vi "configUI.vi"() -> ()   [LabVIEW 2017, in "ActiveFrontEndModule editor node.lvclass"]
doc: "All child modules share this same UI. The UI allows for the configuration of Channels, Parameters, and Error Handling."
uses:
  ActiveFrontEndModule editor node.lvclass
  <vilib>/NI/Configuration Framework/Node/NodeRef.ctl
  <vilib>/NI/Configuration Framework/Node/NISE_CEF_Node.lvclass
  <vilib>/NI/AMC/Message Queue.ctl
  <vilib>/NI/AMC/Message.ctl
  <vilib>/NI/Tools/Keyed Array/KeyedArray.ctl
  <vilib>/NI/Configuration Framework/Node/UserEventRef.ctl
  <vilib>/NI/Configuration Framework/Controls/EventCluster.ctl
  <vilib>/NI/DCAF/Tag Editor Core/control module/configuration/error classification setting.ctl
  <vilib>/NI/Tag Bus Module Framework/runtime/error classification.ctl
  <vilib>/NI/Configuration Framework/Node/RefreshUIEvent.ctl
  <vilib>/NI/Configuration Framework/Node/CacheState.ctl
  <vilib>/NI/Configuration Framework/Node/StopEvent.ctl
  <vilib>/NI/Configuration Framework/Node/NodeChangeEvent.ctl
  <vilib>/NI/DCAF/Tag Editor Core/Table API/Available Tag Menu/channel action event.ctl
  <vilib>/NI/DCAF/Tag Editor Core/Table API/Available Tag Menu/dialog output action.ctl
  <vilib>/NI/Tag Bus Module Framework/channel/TBM channel.lvclass
  <vilib>/NI/Tag Bus/tag/tag descriptor.lvclass
  <vilib>/NI/DCAF/Tag Editor Core/Table API/Table Manager/Call Back Ref Type Def.ctl
  <vilib>/NI/DCAF/Tag Editor Core/Configuration Editor/Classes/Engine Parent/Engine Parent Editor Node.lvclass
  <vilib>/NI/DCAF/Tag Editor Core/Configuration Editor/Classes/Module editor node/module editor node.lvclass
  C:/Program Files (x86)/National Instruments/LabVIEW 2017/vi.lib/NI/Configuration Framework/serializable node/NISE_CEF_serializable node.lvclass
  <vilib>/NI/PowerElectronicsControl/ActiveFrontEnd/AFE/PI_Settings.ctl
  <vilib>/rvi/Analysis/control/PID/Typedef/niFpgaPID_PIGains.ctl
  <vilib>/rvi/Analysis/control/PID/Typedef/niFpgaPID_OutputRange.ctl
  <vilib>/NI/PowerElectronicsControl/ActiveFrontEnd/AFE/Parameters.ctl
  <vilib>/NI/PowerElectronicsControl/ActiveFrontEnd/AFE/Mode.ctl
  <vilib>/NI/DCAF/Tag Editor Core/Table API/Table Manager/references.ctl
  <vilib>/NI/DCAF/Tag Editor Core/Table API/Table Manager/Menu Definition.ctl
  <vilib>/NI/DCAF/Tag Editor Core/Table API/Table Manager/Menu Options.ctl
  <vilib>/NI/DCAF/Tag Editor Core/control module/configuration/control module configuration.lvclass
  C:/Program Files (x86)/National Instruments/LabVIEW 2017/vi.lib/NI/Configuration Framework/serializable configuration/NISE_CEF_serializable configuration.lvclass
  <vilib>/NI/DCAF/Tag Editor Core/control module/editor node/control module editor.lvclass
  C:/Program Files (x86)/National Instruments/LabVIEW 2017/vi.lib/NI/DCAF/Tag Editor Core/Configuration Editor/Classes/Module editor node/module editor node.lvclass
  module/configuration/ActiveFrontEndModule configuration.lvclass
  C:/Program Files (x86)/National Instruments/LabVIEW 2017/vi.lib/NI/DCAF/Tag Editor Core/control module/configuration/control module configuration.lvclass
  C:/Program Files (x86)/National Instruments/LabVIEW 2017/vi.lib/NI/Tag Bus Module Framework/module configuration/TBM module configuration.lvclass
  module/configuration/ActiveFrontEndModule configuration.lvclass/ActiveFrontEndModule configuration.ctl
  <vilib>/NI/DCAF/Tag Editor Core/control module/configuration/control module configuration.lvclass/control module configuration.ctl
  <vilib>/NI/Configuration Framework/serializable configuration/NISE_CEF_serializable configuration.lvclass/NISE_CEF_serializable configuration.ctl
  <vilib>/NI/Tag Bus Module Framework/channel/channel classification.ctl
  module/configuration/Read ID_to_VD.vi
  module/configuration/Read IQ_to_VQ.vi
  module/configuration/Read VDCLinkToPower.vi
  module/configuration/Read Parameters.vi
  module/configuration/Write VDCLinkToPower.vi
  module/configuration/Write ID_to_VD.vi
  module/configuration/Write IQ_to_VQ.vi
  module/configuration/Write Parameters.vi
  <vilib>/NI/DCAF/Tag Editor Core/control module/configuration/Write error classifications.vi
  <vilib>/NI/Tag Bus Module Framework/module configuration/TBM module configuration.lvclass
  <vilib>/NI/DCAF/Tag Editor Core/Configuration Editor/Classes/Module editor node/Read Module Configuration.vi
  <vilib>/NI/DCAF/Tag Editor Core/control module/editor node/read fixed channel configuration.vi
  <vilib>/NI/DCAF/Tag Editor Core/Configuration Editor/Classes/Module editor node/Write Module Configuration.vi
  <vilib>/Utility/LVClass/Get LV Class Name.vi
  <vilib>/NI/Configuration Framework/error generator/NISE_error generator.vi
  <vilib>/NI/Configuration Framework/serializable configuration/NISE_CEF_serializable configuration.lvclass
  <vilib>/NI/DCAF/Tag Editor Core/Table API/Listbox/Multi Column Listbox.lvclass
  <vilib>/NI/Configuration Framework/NISE_CEF_TreeControl.lvlib
  <vilib>/NI/DCAF/Tag Editor Core/Table API/Table Manager.lvlib
  <vilib>/NI/DCAF UI Toolkit/Controls/DCAF UI Elements.lvlib
  <vilib>/NI/Tools/Keyed Array/Tools_KeyedArray.lvlib
  <vilib>/NI/AMC/AMC.lvlib
  <vilib>/NI/DCAF/Tag Editor Core/Table API/Table Manager/Table Manager.lvclass
  <vilib>/NI/Tag Bus Module Framework/runtime/TBM module execution interface.lvclass
  <vilib>/NI/PowerElectronicsControl/ActiveFrontEnd/AFE/ActiveFrontEnd.lvlib
panel:
  in  "Enum":i32
  in  "user event out":refnum<user-event>
  in  "Top Level Tab Control":T1(tab)
  in  "ID_to_VD":T2={"gains"={"proportional gain"=0.0, "integral gain"=0.0}, "output range"={"output high (Inf)"=inf, "output low (-Inf)"=-inf}, "PI_state"=enum."idle", "reset"=FALSE, "manual"=0.0} {"gains"."proportional gain" step=0.125}
  in  "IQ_to_VQ":T2={"gains"={"proportional gain"=0.0, "integral gain"=0.0}, "output range"={"output high (Inf)"=inf, "output low (-Inf)"=-inf}, "PI_state"=enum."idle", "reset"=FALSE, "manual"=0.0} {"gains"."proportional gain" step=0.125}
  in  "VDCLinkToPower":T2={"gains"={"proportional gain"=0.0, "integral gain"=0.0}, "output range"={"output high (Inf)"=inf, "output low (-Inf)"=-inf}, "PI_state"=enum."idle", "reset"=FALSE, "manual"=0.0} {"gains"."proportional gain" step=0.125}
  in  "Initial Parameters":T5
  in  "Channels Listbox":i32(listbox)
  in  "mapall":bool
  in  "mapwriters":bool
  in  "Parameters Listbox":i32(listbox)
  in  "error classifications":T7[](array[typedef])
  in  "node change":T9
  in  "stop event":T10
  in  "cache state":T11
  in  "refresh UI":T12
  in  "user event":T13
  in  "main queue":T14
  in  "node ref":T15
  # "(Single-Click to Edit)"
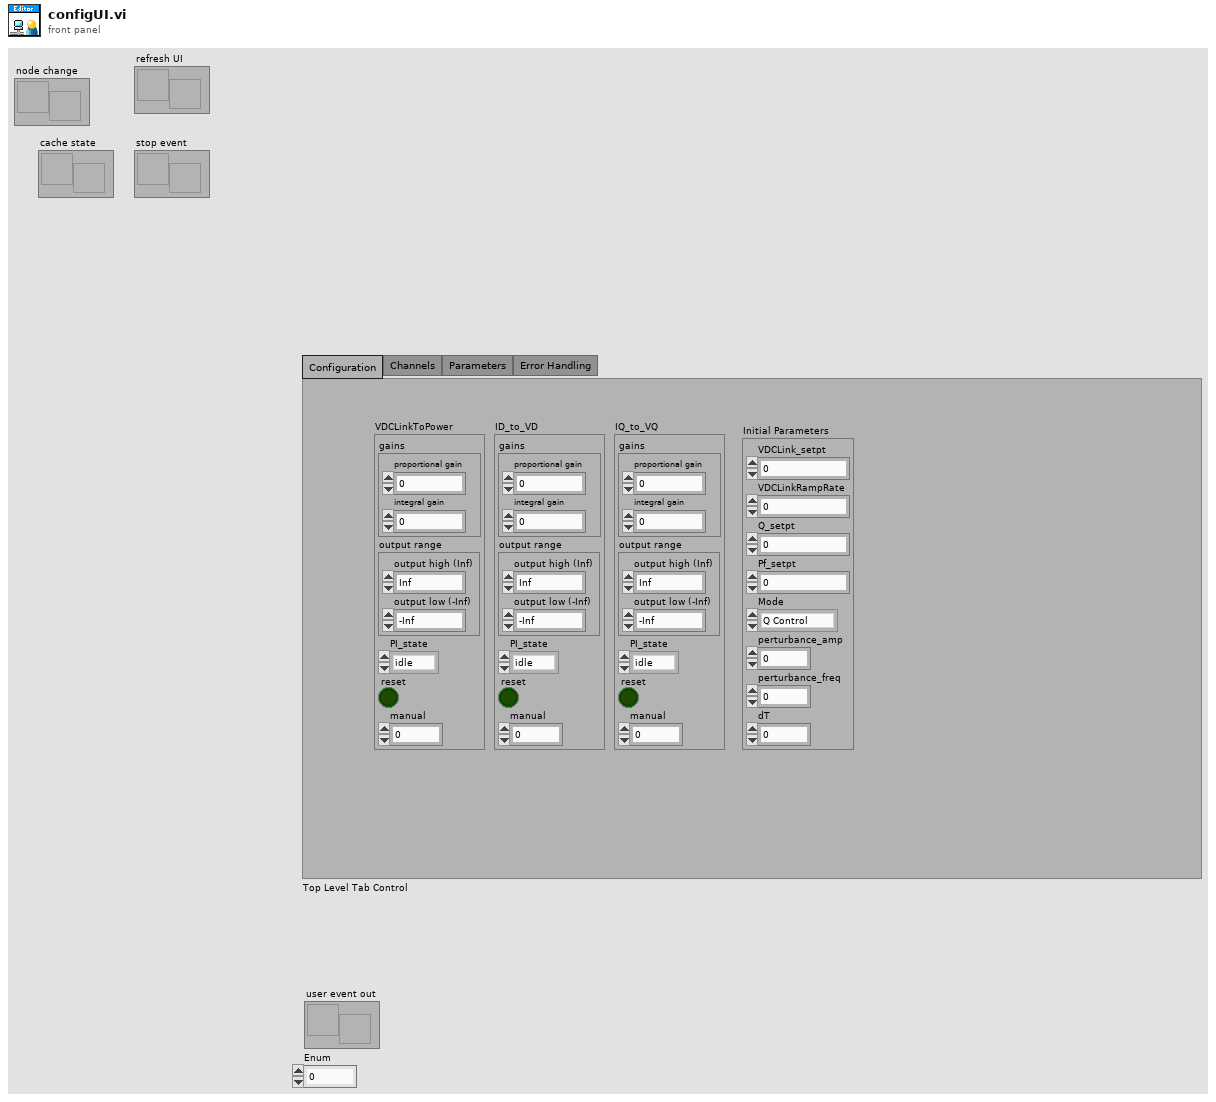
[diagram p1: front panel]
types:
  T1 = enum32{"Configuration", "Channels", "Parameters", "Error Handling"}
  T2 = typedef "ActiveFrontEnd.lvlib/PI_Settings.ctl" = cluster{"gains":T3, "output range":T4, "PI_state":enum8{"idle", "normal", "manual", "perturbance"}, "reset":bool, "manual":sgl}
  T3 = typedef "niFpgaPID_PIGains.ctl" = cluster{"proportional gain":sgl, "integral gain":sgl}
  T4 = typedef "niFpgaPID_OutputRange.ctl" = cluster{"output high (Inf)":sgl, "output low (-Inf)":sgl}
  T5 = typedef "ActiveFrontEnd.lvlib/Parameters.ctl" = cluster{"VDCLink_setpt":sgl, "VDCLinkRampRate":sgl, "Q_setpt":sgl, "Pf_setpt":sgl, "Mode":T6, "perturbance_amp":sgl, "perturbance_freq":sgl, "dT":sgl}
  T6 = typedef "ActiveFrontEnd.lvlib/Mode.ctl" = enum16{"Q Control", "Pf Control"}
  T7 = typedef "control module configuration.lvclass/error classification setting.ctl" = cluster{"code":i32, "error classification":T8}
  T8 = typedef "TBM module execution interface.lvclass/error classification.ctl" = enum16{"unknown", "none", "trivial", "recoverable", "critical"}
  T9 = typedef "NISE_CEF_Node.lvclass/NodeChangeEvent.ctl" = refnum<user-event>
  T10 = typedef "NISE_CEF_Node.lvclass/StopEvent.ctl" = refnum<user-event>
  T11 = typedef "NISE_CEF_Node.lvclass/CacheState.ctl" = refnum<user-event>
  T12 = typedef "NISE_CEF_Node.lvclass/RefreshUIEvent.ctl" = refnum<user-event>
  T13 = typedef "NISE_CEF_Node.lvclass/UserEventRef.ctl" = refnum<user-event>
  T14 = typedef "AMC.lvlib/Message Queue.ctl" = refnum<queue>
  T15 = typedef "NISE_CEF_Node.lvclass/NodeRef.ctl" = refnum<data-value>
  T16 = typedef "Table Manager.lvlib/Table Manager.lvclass/Menu Definition.ctl" = cluster{"Menu Name":string, "Menu Options":T17}
  T17 = typedef "Table Manager.lvlib/Table Manager.lvclass/Menu Options.ctl" = enum16{"Always Show", "Show When Used", "Show When Empty"}
  T18 = typedef "Table Manager.lvlib/Table Manager.lvclass/references.ctl" = cluster{"stop event":T10, "refresh UI":T12, "cache state":T11, "node change":T9, "user event out":refnum<user-event>, "main queue":T14, "user event":T13}
  T19 = typedef "Table Manager.lvlib/Column.lvclass/Column Descriptor.ctl" = cluster{"name":string, "caption":string, "Column Type":T20, "Params":string, "AutoSizeMode":i32, "FillWeight":sgl, "MinWidth":u32, "tooltip":string, "Enum Reference":refnum<vi>, "Channel suffix":string, "Read Only":bool, "Call Back VI":T21, "DT Dependency":i32, "name dependency":i32, "data type":T22, "Custom Column":refnum<class "Column.lvclass">}
  T20 = typedef "Table Manager.lvlib/Column.lvclass/Column Type.ctl" = enum16{"String", "Mapping", "Enum", "Custom"}
  T21 = typedef "Table Manager.lvlib/Table Manager.lvclass/Call Back Ref Type Def.ctl" = refnum<vi>
  T22 = typedef "tag bus.lvlib/tag descriptor.lvclass/Data Type.ctl" = enum16{"Double", "Single", "I64", "I32", "I16", "I8", "U64", "U32", "U16", "U8", "Boolean", "String", "Array of Double", "Array of Single", "Array of I64", "Array of I32", "Array of I16", "Array of I8", "Array of U64", "Array of U32", "Array of U16", "Array of U8", "Array of Boolean", "Array of String"}
  T23 = typedef "Table Manager.lvlib/Table Manager.lvclass/object ref.ctl" = cluster{"engine":refnum<data-value>, "Node Ref":refnum<data-value>}
  T24 = typedef "Table Manager.lvlib/Table Manager.lvclass/Table Events.ctl" = cluster{"Menu Selection":refnum<user-event>}
  T25 = typedef "NISE_CEF_TreeControl.lvlib/EventCluster.ctl" = cluster{"command":string, "data":string}
  T26 = typedef "TBM channel.lvclass/channel classification.ctl" = enum16{"input data", "output data", "processing parameter", "processing result"}
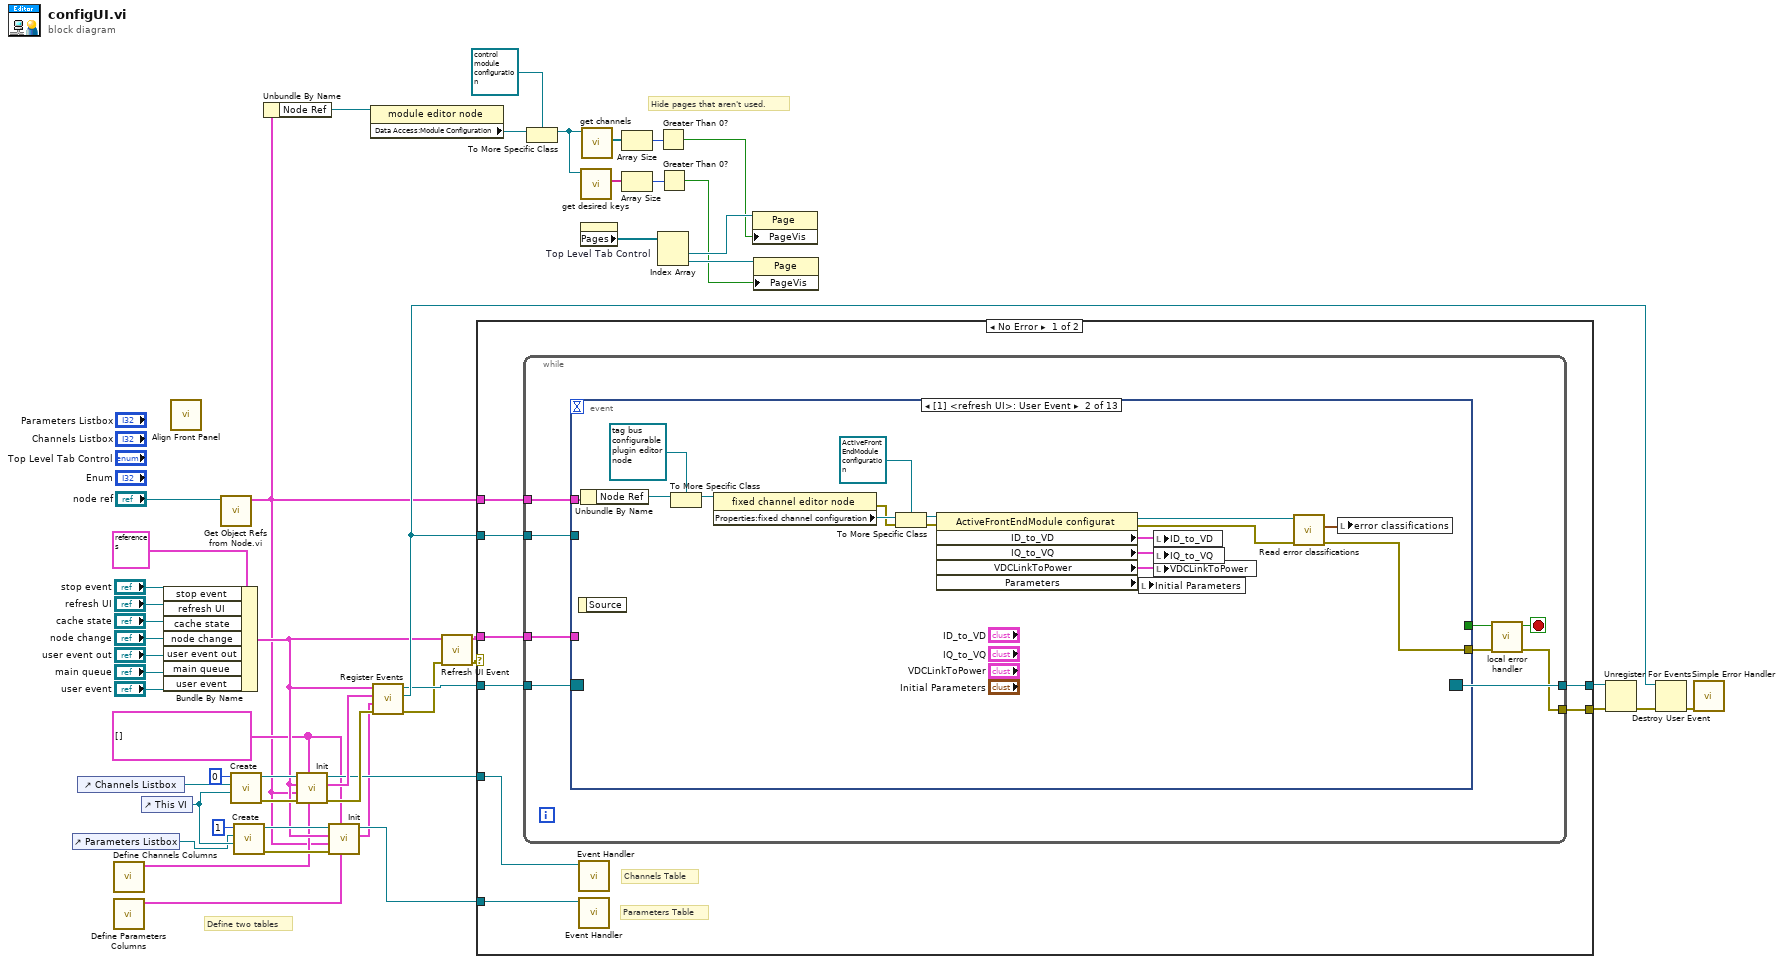
[diagram p0: block diagram]
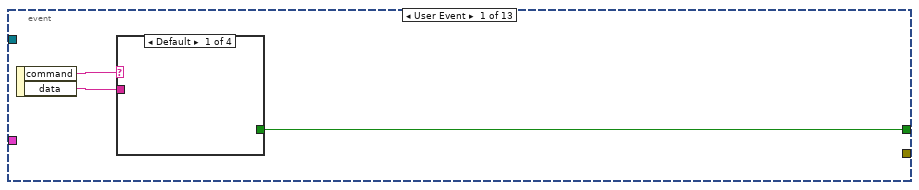
[diagram p2: hidden frame]
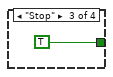
[diagram p4: hidden frame]
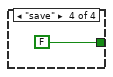
[diagram p5: hidden frame]
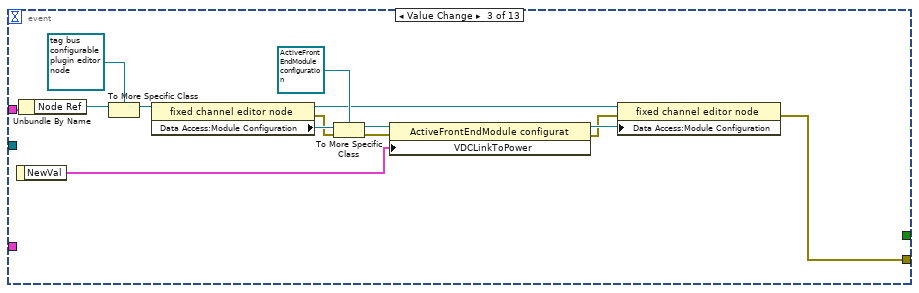
[diagram p6: hidden frame]
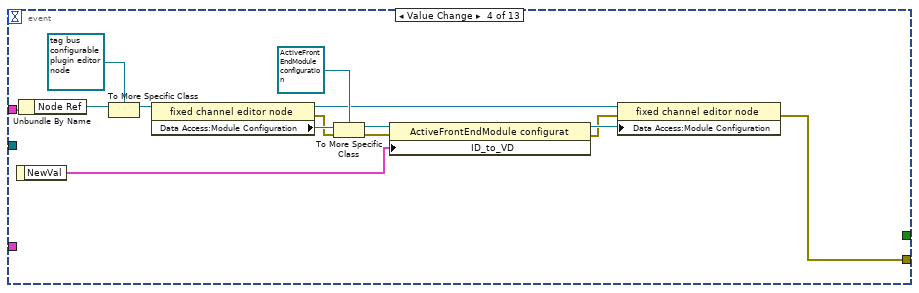
[diagram p7: hidden frame]
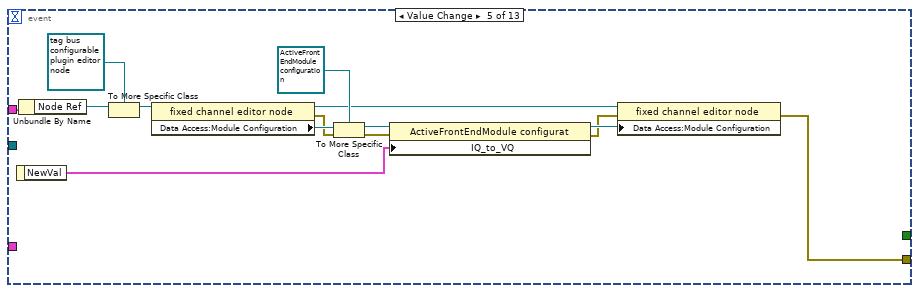
[diagram p8: hidden frame]
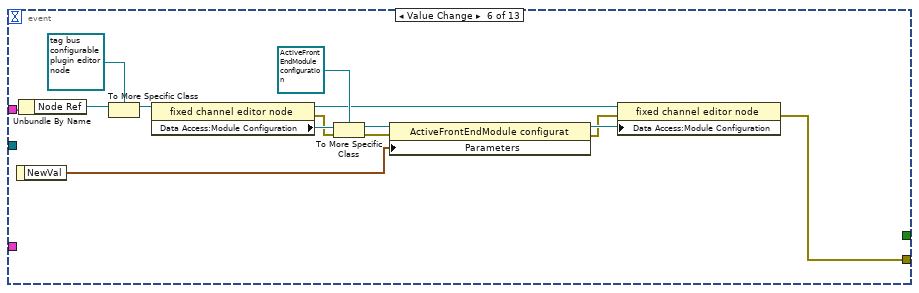
[diagram p9: hidden frame]
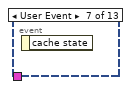
[diagram p10: hidden frame]
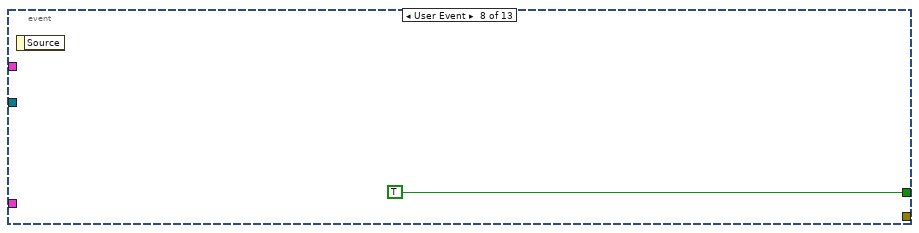
[diagram p11: hidden frame]
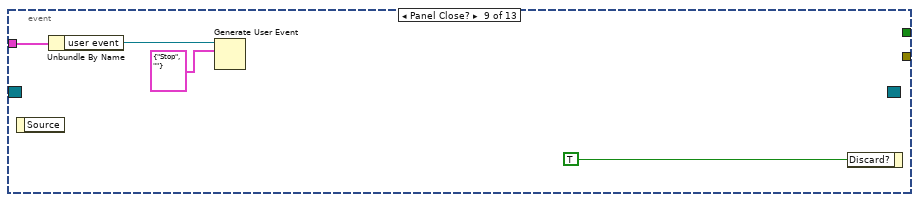
[diagram p12: hidden frame]
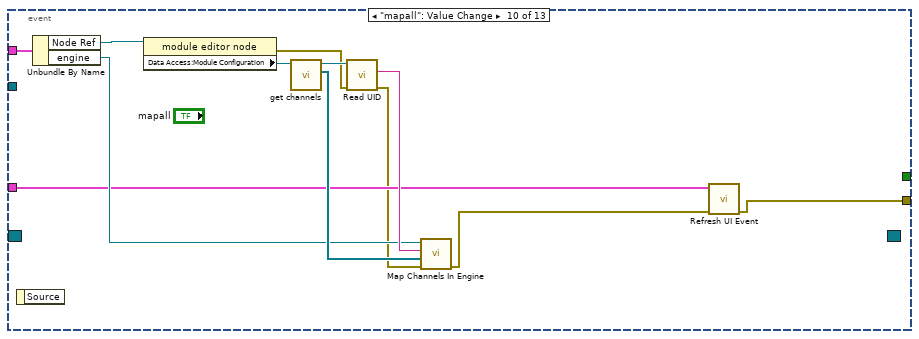
[diagram p13: hidden frame]
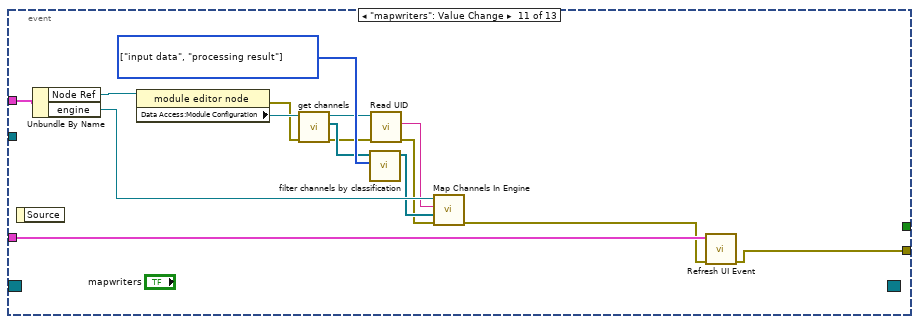
[diagram p14: hidden frame]
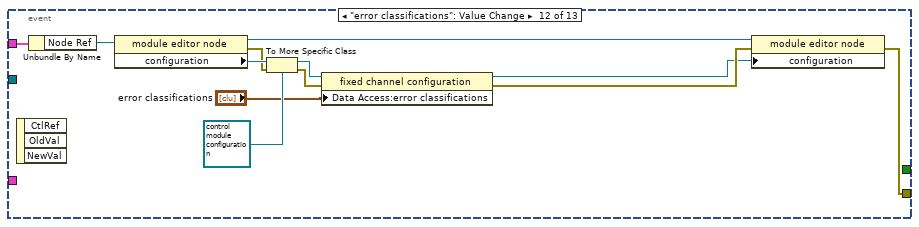
[diagram p15: hidden frame]
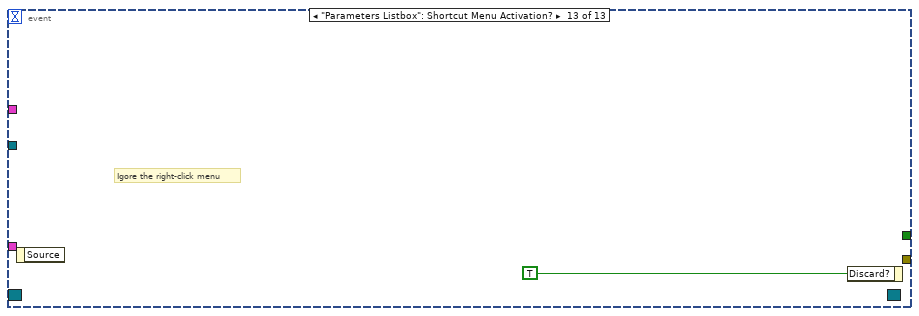
[diagram p16: hidden frame]
diagram:
  w15 = T16[] [] ("Right-Click Menu")
  # "Define two tables"
  # "Hide pages that aren't used."
  n1 = control-ref of="Parameters Listbox"() -> (w18:refnum<vi>)
  n2 = control-ref of="Channels Listbox"() -> (w26:refnum<vi>)
  n3 = call <vilib>:"Define Channels Columns.vi"() -> ("Column Descriptors"=w17:T19[])  [unwired: 11 in]
  n4 = call <vilib>:"Define Parameters Columns.vi"() -> ("Column Descriptors"=w16:T19[])  [unwired: 11 in]
  n5 = control-ref of="This VI"() -> (w22:refnum<vi>)
  n6 = Bundle By Name(cluster=T18 {"stop event"=refnum, "refresh UI"=refnum, "cache state"=refnum, "node change"=refnum, "user event out"=refnum, "main queue"=refnum, "user event"=refnum} ("Event References"), "stop event"="stop event", "refresh UI"="refresh UI", "cache state"="cache state", "node change"="node change", "user event out"="user event out", "main queue"="main queue", "user event"="user event") -> (w19:T18)
  n7 = call <vilib>:"Align Front Panel.vi"() -> ()  [unwired: 10 in, 2 out]
  n8 = call <vilib>:"Get Object Refs from Node.vi.vi"("node ref"="node ref") -> ("Node object refs"=w7:T23)  [unwired: 9 in, 1 out]
  n9 = call <vilib>:"Create.vi"("Top VI"=w22, "Listbox"=w26, "Index"=0) -> ("error out"=w29:errorcluster, "reference out"=w30:refnum<class "Multi Column Listbox.lvclass">)  [unwired: 7 in]
  n10 = call <vilib>:"Create.vi"("Top VI"=w22, "Listbox"=w18, "Index"=1) -> ("error out"=w25:errorcluster, "reference out"=w24:refnum<class "Multi Column Listbox.lvclass">)  [unwired: 7 in]
  n11 = Unbundle By Name(w7) -> ("Node Ref"=w5:refnum<data-value>)
  n12 = call-dynamic "Init.vi"("Column Descriptors"=w17, "Right-Click Menu"=w15, "error in (no error)"=w29, "Node object refs"=w7, "Event References"=w19, "Multi Column Listbox in"=w30) -> ("error out"=w28:errorcluster, "Table Events"=w40:T24, "Multi Column Listbox out"=w27:refnum<class "Multi Column Listbox.lvclass">)  [unwired: 3 in]
  n13 = call-dynamic "Init.vi"("Column Descriptors"=w16, "Right-Click Menu"=w15, "error in (no error)"=w25, "Node object refs"=w7, "Event References"=w19, "Multi Column Listbox in"=w24) -> ("Table Events"=w20:T24, "Multi Column Listbox out"=w21:refnum<class "Multi Column Listbox.lvclass">)  [unwired: 3 in, 1 out]
  n14 = property class="module editor node"(reference=w5) -> ("Data Access:Module Configuration"=w6:refnum<class "TBM module configuration.lvclass">)  [unwired: 1 in, 2 out]
  n15 = call <vilib>:"Register Events.vi"("error in (no error)"=w28, "Parameters Table Events"=w20, "Channels Table Events"=w40, "Event References"=w19) -> ("error out"=w33:errorcluster, "Channel Action"=w39:refnum<user-event>, "Event Registration Refnum"=w38:refnum<event-registration>)  [unwired: 5 in]
  n16 = call <vilib>:"Refresh UI Event.vi"("error in (no error)"=w33, "Event References"=w19) -> ("error out"=w34:errorcluster, "Event References out"=w32:T18)  [unwired: 8 in]
  n17 = case shown="No Error" w34 {
    selector: w34 -> [_ w191]
    tunnel: w38 -> [w58 w190]
    tunnel: [w57 w190] -> w50
    tunnel: [w55 w191] -> w49
    tunnel: w39 -> [w56 _]
    tunnel: w7 -> [w54 _]
    tunnel: w32 -> [w53 _]
    tunnel: w27 -> [w52 _]
    tunnel: w21 -> [w51 _]
    frame No Error {
      # "Parameters Table"
      # "Channels Table"
      n18 = while {
        tunnel: w58 -> [w67]
        tunnel: [w66] -> w57
        tunnel: w56 -> [w65]
        tunnel: [w61] -> w55
        tunnel: w54 -> [w60]
        tunnel: w53 -> [w59]
        stop <- w63 stop-if-true
        n19 = event shown="[1] <refresh UI>: User Event" {
          selector: w67 -> [_ _ _ _ _ _ _ _ _ _ _ _ _]
          dyn-events: [_ _ _ _ _ _ _ _ _ _ _ _ _] -> w66
          timeout: _ -> [_ _ _ _ _ _ _ _ _ _ _ _ _]
          tunnel: [w70 _ _ _ _ _ _ TRUE _ _ _ _ _] -> w64
          tunnel: [_ w86 w91 w105 w119 w133 _ _ _ w156 w172 w188 _] -> w62
          tunnel: w65 -> [_ _ _ _ _ _ _ _ _ _ _ _ _]
          tunnel: w60 -> [_ w89 w103 w117 w131 w145 _ _ _ w160 w173 w187 _]
          tunnel: w59 -> [_ _ _ _ _ _ _ _ w148 w155 w171 _ _]
          event User Event {
            n20 = event-data() -> ("command"=w69:string, "data"=w68:string)  [unwired: 1 in]
            n21 = case shown="Default" w69 {
              tunnel: [_ _ TRUE FALSE] -> w70
              tunnel: w68 -> [_ _ _ _]
              frame Default {
              }
              frame "Refresh" {
              }
              frame "Stop" {
              }
              frame "save" {
              }
            }
          }
          event User Event {
            n22 = event-data() -> ()  [unwired: 1 in, 1 out]
            n23 = Unbundle By Name(w89) -> ("Node Ref"=w87:refnum<data-value>)
            n24 = To More Specific Class(target class=refnum<data-value> refnum ("data value reference"), reference=w87) -> (specific class reference=w85:refnum<data-value>)  [unwired: 1 in, 1 out]
            n25 = property class="fixed channel editor node"(reference=w85) -> (error out=w82:errorcluster, "Properties:fixed channel configuration"=w83:refnum<class "control module configuration.lvclass">)  [unwired: 1 in, 1 out]
            n26 = To More Specific Class(target class=refnum<class "ActiveFrontEndModule configuration.lvclass"> refnum ("ActiveFrontEndModule configuration"), reference=w83, error in=w82) -> (specific class reference=w80:refnum<class "ActiveFrontEndModule configuration.lvclass">, error out=w78:errorcluster)
            n27 = property class="ActiveFrontEndModule configurat"(reference=w80, error in=w78) -> (reference out=w79:refnum<class "ActiveFrontEndModule configuration.lvclass">, error out=w77:errorcluster, "ID_to_VD"=w76:T2, "IQ_to_VQ"=w75:T2, "VDCLinkToPower"=w74:T2, "Parameters"=w73:T5)
            n28 = local write "Initial Parameters"(w73) -> ()
            n29 = local write "ID_to_VD"(w76) -> ()
            n30 = local write "IQ_to_VQ"(w75) -> ()
            n31 = local write "VDCLinkToPower"(w74) -> ()
            n32 = call <vilib>:"Read error classifications.vi"("error in"=w77, "control module configuration in"=w79) -> ("error out"=w86:errorcluster, "error classifications"=w84:T7[])  [unwired: 7 in, 1 out]
            n33 = local write "error classifications"(w84) -> ()
          }
          event Value Change {
            n34 = event-data() -> ("NewVal"=w90:T2)  [unwired: 1 in]
            n35 = Unbundle By Name(w103) -> ("Node Ref"=w101:refnum<data-value>)
            n36 = To More Specific Class(target class=refnum<data-value> refnum ("data value reference"), reference=w101) -> (specific class reference=w100:refnum<data-value>)  [unwired: 1 in, 1 out]
            n37 = property class="fixed channel editor node"(reference=w100) -> (reference out=w94:refnum<data-value>, error out=w98:errorcluster, "Data Access:Module Configuration"=w99:refnum<class "TBM module configuration.lvclass">)  [unwired: 1 in]
            n38 = To More Specific Class(target class=refnum<class "ActiveFrontEndModule configuration.lvclass"> refnum ("ActiveFrontEndModule configuration"), reference=w99, error in=w98) -> (specific class reference=w96:refnum<class "ActiveFrontEndModule configuration.lvclass">, error out=w95:errorcluster)
            n39 = property class="ActiveFrontEndModule configurat"(reference=w96, error in=w95, "VDCLinkToPower"=w90) -> (reference out=w93:refnum<class "ActiveFrontEndModule configuration.lvclass">, error out=w92:errorcluster)
            n40 = property class="fixed channel editor node"(reference=w94, error in=w92, "Data Access:Module Configuration"=w93) -> (error out=w91:errorcluster)  [unwired: 1 out]
          }
          event Value Change {
            n41 = event-data() -> ("NewVal"=w104:T2)  [unwired: 1 in]
            n42 = Unbundle By Name(w117) -> ("Node Ref"=w115:refnum<data-value>)
            n43 = To More Specific Class(target class=refnum<data-value> refnum ("data value reference"), reference=w115) -> (specific class reference=w114:refnum<data-value>)  [unwired: 1 in, 1 out]
            n44 = property class="fixed channel editor node"(reference=w114) -> (reference out=w108:refnum<data-value>, error out=w112:errorcluster, "Data Access:Module Configuration"=w113:refnum<class "TBM module configuration.lvclass">)  [unwired: 1 in]
            n45 = To More Specific Class(target class=refnum<class "ActiveFrontEndModule configuration.lvclass"> refnum ("ActiveFrontEndModule configuration"), reference=w113, error in=w112) -> (specific class reference=w110:refnum<class "ActiveFrontEndModule configuration.lvclass">, error out=w109:errorcluster)
            n46 = property class="ActiveFrontEndModule configurat"(reference=w110, error in=w109, "ID_to_VD"=w104) -> (reference out=w107:refnum<class "ActiveFrontEndModule configuration.lvclass">, error out=w106:errorcluster)
            n47 = property class="fixed channel editor node"(reference=w108, error in=w106, "Data Access:Module Configuration"=w107) -> (error out=w105:errorcluster)  [unwired: 1 out]
          }
          event Value Change {
            n48 = event-data() -> ("NewVal"=w118:T2)  [unwired: 1 in]
            n49 = Unbundle By Name(w131) -> ("Node Ref"=w129:refnum<data-value>)
            n50 = To More Specific Class(target class=refnum<data-value> refnum ("data value reference"), reference=w129) -> (specific class reference=w128:refnum<data-value>)  [unwired: 1 in, 1 out]
            n51 = property class="fixed channel editor node"(reference=w128) -> (reference out=w122:refnum<data-value>, error out=w126:errorcluster, "Data Access:Module Configuration"=w127:refnum<class "TBM module configuration.lvclass">)  [unwired: 1 in]
            n52 = To More Specific Class(target class=refnum<class "ActiveFrontEndModule configuration.lvclass"> refnum ("ActiveFrontEndModule configuration"), reference=w127, error in=w126) -> (specific class reference=w124:refnum<class "ActiveFrontEndModule configuration.lvclass">, error out=w123:errorcluster)
            n53 = property class="ActiveFrontEndModule configurat"(reference=w124, error in=w123, "IQ_to_VQ"=w118) -> (reference out=w121:refnum<class "ActiveFrontEndModule configuration.lvclass">, error out=w120:errorcluster)
            n54 = property class="fixed channel editor node"(reference=w122, error in=w120, "Data Access:Module Configuration"=w121) -> (error out=w119:errorcluster)  [unwired: 1 out]
          }
          event Value Change {
            n55 = event-data() -> ("NewVal"=w132:T5)  [unwired: 1 in]
            n56 = Unbundle By Name(w145) -> ("Node Ref"=w143:refnum<data-value>)
            n57 = To More Specific Class(target class=refnum<data-value> refnum ("data value reference"), reference=w143) -> (specific class reference=w142:refnum<data-value>)  [unwired: 1 in, 1 out]
            n58 = property class="fixed channel editor node"(reference=w142) -> (reference out=w136:refnum<data-value>, error out=w140:errorcluster, "Data Access:Module Configuration"=w141:refnum<class "TBM module configuration.lvclass">)  [unwired: 1 in]
            n59 = To More Specific Class(target class=refnum<class "ActiveFrontEndModule configuration.lvclass"> refnum ("ActiveFrontEndModule configuration"), reference=w141, error in=w140) -> (specific class reference=w138:refnum<class "ActiveFrontEndModule configuration.lvclass">, error out=w137:errorcluster)
            n60 = property class="ActiveFrontEndModule configurat"(reference=w138, error in=w137, "Parameters"=w132) -> (reference out=w135:refnum<class "ActiveFrontEndModule configuration.lvclass">, error out=w134:errorcluster)
            n61 = property class="fixed channel editor node"(reference=w136, error in=w134, "Data Access:Module Configuration"=w135) -> (error out=w133:errorcluster)  [unwired: 1 out]
          }
          event User Event {
            n62 = event-data() -> ()  [unwired: 1 in, 1 out]
          }
          event User Event {
            n63 = event-data() -> ()  [unwired: 1 in, 1 out]
          }
          event Panel Close? {
            n64 = event-data() -> ()  [unwired: 1 in, 1 out]
            n65 = Unbundle By Name(w148) -> ("user event"=w147:T13)
            n66 = Generate User Event(user event=w147, event data cluster=T25 {"command"="Stop", "data"=""} ("event data")) -> ()  [unwired: 2 in, 2 out]
            n67 = event-data("Discard?"=TRUE) -> ()  [unwired: 1 in, 1 out]
          }
          event "mapall": Value Change {
            n68 = event-data() -> ()  [unwired: 1 in, 1 out]
            n69 = Unbundle By Name(w160) -> ("Node Ref"=w159:refnum<data-value>, "engine"=w158:refnum<data-value>)
            n70 = property class="module editor node"(reference=w159) -> (error out=w152:errorcluster, "Data Access:Module Configuration"=w154:refnum<class "TBM module configuration.lvclass">)  [unwired: 1 in, 1 out]
            n71 = call-dynamic "get channels.vi"("module configuration in"=w154) -> ("channels"=w162:refnum<class "TBM channel.lvclass">[], "module configuration out"=w153:refnum<class "TBM module configuration.lvclass">)  [unwired: 9 in]
            n72 = call <vilib>:"Read UID.vi"("error in"=w152, "configuration in"=w153) -> ("error out"=w151:errorcluster, "instance id"=w161:string)  [unwired: 7 in, 1 out]
            n73 = call <vilib>:"Map Channels In Engine.vi"("error in (no error)"=w151, "channels"=w162, "instance id"=w161, "Engine DVR"=w158) -> ("error out"=w157:errorcluster)  [unwired: 7 in]
            n74 = call <vilib>:"Refresh UI Event.vi"("error in (no error)"=w157, "Event References"=w155) -> ("error out"=w156:errorcluster)  [unwired: 8 in, 1 out]
          }
          event "mapwriters": Value Change {
            w176 = T26[] [enum."input data", enum."processing result"] items=["input data", "output data", "processing parameter", "processing result"] ("allowed classifications")
            n75 = event-data() -> ()  [unwired: 1 in, 1 out]
            n76 = Unbundle By Name(w173) -> ("Node Ref"=w174:refnum<data-value>, "engine"=w170:refnum<data-value>)
            n77 = property class="module editor node"(reference=w174) -> (error out=w163:errorcluster, "Data Access:Module Configuration"=w165:refnum<class "TBM module configuration.lvclass">)  [unwired: 1 in, 1 out]
            n78 = call-dynamic "get channels.vi"("module configuration in"=w165) -> ("channels"=w175:refnum<class "TBM channel.lvclass">[], "module configuration out"=w164:refnum<class "TBM module configuration.lvclass">)  [unwired: 9 in]
            n79 = call <vilib>:"filter channels by classification.vi"("allowed classifications"=w176, "channels in"=w175) -> ("channels out"=w168:refnum<class "TBM channel.lvclass">[])  [unwired: 9 in]
            n80 = call <vilib>:"Read UID.vi"("error in"=w163, "configuration in"=w164) -> ("error out"=w167:errorcluster, "instance id"=w169:string)  [unwired: 7 in, 1 out]
            n81 = call <vilib>:"Map Channels In Engine.vi"("error in (no error)"=w167, "channels"=w168, "instance id"=w169, "Engine DVR"=w170) -> ("error out"=w166:errorcluster)  [unwired: 7 in]
            n82 = call <vilib>:"Refresh UI Event.vi"("error in (no error)"=w166, "Event References"=w171) -> ("error out"=w172:errorcluster)  [unwired: 8 in, 1 out]
          }
          event "error classifications": Value Change {
            n83 = event-data() -> ()  [unwired: 1 in, 3 out]
            n84 = Unbundle By Name(w187) -> ("Node Ref"=w182:refnum<data-value>)
            n85 = property class="module editor node"(reference=w182) -> (reference out=w186:refnum<data-value>, error out=w178:errorcluster, "configuration"=w181:refnum<class "NISE_CEF_serializable configuration.lvclass">)  [unwired: 1 in]
            n86 = To More Specific Class(target class=refnum<class "control module configuration.lvclass"> refnum ("fixed channel configuration"), reference=w181, error in=w178) -> (specific class reference=w183:refnum<class "control module configuration.lvclass">, error out=w177:errorcluster)
            n87 = property class="fixed channel configuration"(reference=w183, error in=w177, "Data Access:error classifications"="error classifications") -> (reference out=w184:refnum<class "control module configuration.lvclass">, error out=w185:errorcluster)
            n88 = property class="module editor node"(reference=w186, error in=w185, "configuration"=w184) -> (error out=w188:errorcluster)  [unwired: 1 out]
          }
          event "Parameters Listbox": Shortcut Menu Activation? {
            # "Igore the right-click menu"
            n89 = event-data() -> ()  [unwired: 1 in, 1 out]
            n90 = event-data("Discard?"=TRUE) -> ()  [unwired: 1 in, 1 out]
          }
        }
        n91 = call <vilib>:"local error handler.vi"("error in (no error)"=w62, "Stop in"=w64) -> ("error out"=w61:errorcluster, "Stop out"=w63:bool)  [unwired: 8 in]
      }
      n92 = call-dynamic "Event Handler.vi"("Listbox in"=w52) -> ()  [unwired: 9 in, 2 out]
      n93 = call-dynamic "Event Handler.vi"("Listbox in"=w51) -> ()  [unwired: 9 in, 2 out]
    }
    frame Error {
    }
  }
  n94 = To More Specific Class(target class=refnum<class "control module configuration.lvclass"> refnum ("fixed channel configuration"), reference=w6) -> (specific class reference=w3:refnum<class "control module configuration.lvclass">)  [unwired: 1 in, 1 out]
  n95 = call-dynamic "get desired keys.vi"("fixed channel configuration in"=w3) -> ("desired keys"=w11:string[])  [unwired: 8 in, 2 out]
  n96 = property on="Top Level Tab Control" class="TabCtl (strict)"() -> ("Pages"=w8:refnum<vi>[])  [unwired: 2 in, 2 out]
  n97 = call-dynamic "get channels.vi"("fixed channel configuration in"=w3) -> ("channels"=w14:refnum<class "TBM channel.lvclass">[])  [unwired: 9 in, 1 out]
  n98 = Array Size(array=w14) -> (size(s)=w13:i32)
  n99 = Array Size(array=w11) -> (size(s)=w12:i32)
  n100 = Greater Than 0?(x=w13) -> (x > 0?=w2:bool)
  n101 = Index Array(array=w8) -> (element #1=w9:refnum<vi>, element #2=w10:refnum<vi>)  [unwired: 2 in]
  n102 = Greater Than 0?(x=w12) -> (x > 0?=w1:bool)
  n103 = property class="Page"(reference=w9, "PageVis"=w2) -> ()  [unwired: 1 in, 2 out]
  n104 = property class="Page"(reference=w10, "PageVis"=w1) -> ()  [unwired: 1 in, 2 out]
  n105 = Unregister For Events(event registration refnum=w50, error in=w49) -> (error out=w48:errorcluster)
  n106 = Destroy User Event(user event=w39, error in=w48) -> (error out=w47:errorcluster)
  n107 = call <vilib>:"Simple Error Handler.vi"("error in (no error)"=w47) -> ()  [unwired: 4 in, 5 out]
